vi "find number interval.vi"(8 "error in (no error)":errorcluster, 9 "Numeric":dbl, 10 "Array":dbl[](array[numeric]), 11 "Simulated Camera in":refnum<class "Simulated Camera.lvclass">) -> (0 "error out":errorcluster, 2 "index":i32, 3 "Simulated Camera out":refnum<class "Simulated Camera.lvclass">)   [LabVIEW 2018, in "Simulated Camera.lvclass"]
uses:
  Simulated Camera.lvclass
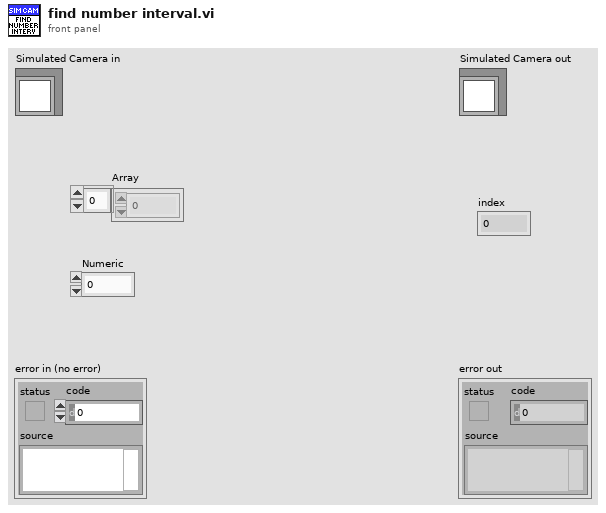
[diagram p1: front panel]
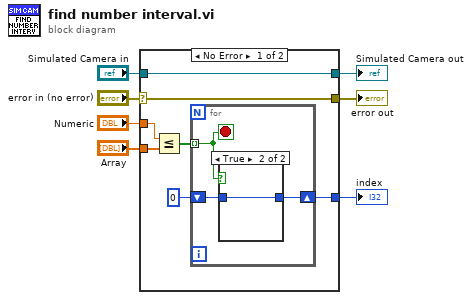
[diagram p0: block diagram]
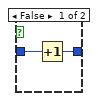
[diagram p2: hidden frame]
diagram:
  n1 = case shown="No Error" "error in (no error)" {
    selector: "error in (no error)" -> [w13 w22]
    tunnel: [w13 w22] -> w6
    tunnel: [w14 w21] -> w4
    tunnel: "Simulated Camera in" -> [w14 w21]
    tunnel: "Array" -> [w8 _]
    tunnel: "Numeric" -> [w9 _]
    tunnel: [w10 _] -> w1
    frame No Error {
      n2 = Less Or Equal?(x=w9, y=w8) -> (x <= y?=w12:bool[])
      n3 = for {
        tunnel: w12 -> [w17] mode=indexing
        shift-right: [w15] -> w10
        shift-left: 0 -> [w16]
        stop <- w17 stop-if-true
        n4 = case shown="True" w17 {
          tunnel: w16 -> [w19 w20]
          tunnel: [w18 w20] -> w15
          frame False {
            n5 = Increment(x=w19) -> (x+1=w18:i32)
          }
          frame True {
          }
        }
      }
    }
    frame Error {
    }
  }
  "error out" <- w6
  "Simulated Camera out" <- w4
  "index" <- w1
